vi "DHE_SetModuleName.vi"(2 "DHE_ModuleName":string) -> ()   [LabVIEW 2016]
uses:
  DHE_GBLDriverVariables.vi
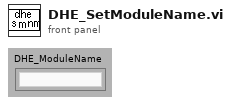
[diagram p1: front panel]
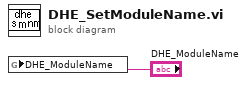
[diagram p0: block diagram]
diagram:
  n1 = global write "DHE_GBLDriverVariables.vi" "DHE_ModuleName"("DHE_ModuleName") -> ()
